vi "solar_voy_def Export (Mods_State).vi"(10 "CMD":enum8{"CMD", "TLM"}(ring), 11 "STATE":T1) -> (3 "STATE_DEF":string)   [LabVIEW 2018]
doc: "This exports a COSMOS state modifier to string."
uses:
  solar_voy_def_ctl MODIFIERS STATE.ctl
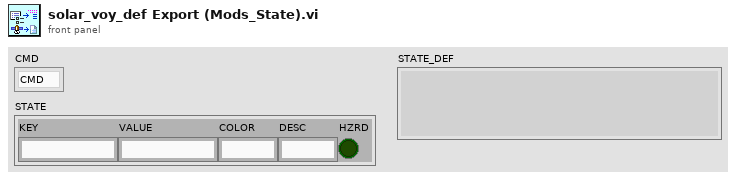
[diagram p1: front panel]
types:
  T1 = typedef "solar_voy_def_ctl MODIFIERS STATE.ctl" = cluster{"KEY":string, "VALUE":string, "COLOR":string, "DESC":string, "HZRD":bool}
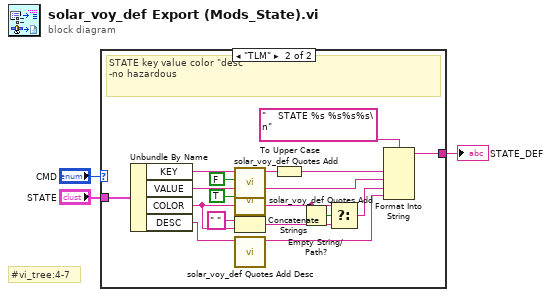
[diagram p0: block diagram]
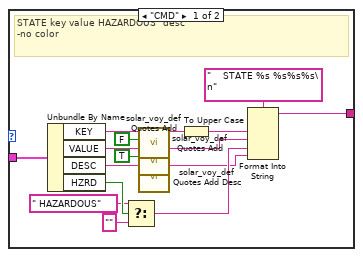
[diagram p2: hidden frame]
diagram:
  # "#vi_tree:4-7"
  n1 = case shown="\"TLM\"" "CMD" {
    tunnel: "STATE" -> [w19 w36]
    tunnel: [w12 w28] -> w2
    frame "CMD" {
      # "STATE key value HAZARDOUS \"desc\"\n-no color"
      n2 = Unbundle By Name(w19) -> ("KEY"=w17:string, "VALUE"=w16:string, "DESC"=w7:string, "HZRD"=w11:bool)
      n3 = Select(t=" HAZARDOUS", s=w11, f="") -> (s? t:f=w8:string)
      n4 = call "solar_voy_def Quotes Add.vi"("Whitespace Only? (F=Always)"=FALSE, "String"=w17) -> ("String with Comments"=w13:string)  [unwired: 9 in]
      n5 = call "solar_voy_def Quotes Add.vi"("Whitespace Only? (F=Always)"=TRUE, "String"=w16) -> ("String with Comments"=w5:string)  [unwired: 9 in]
      n6 = call "solar_voy_def Quotes Add Desc.vi"("Description"=w7) -> ("Description with Comments"=w6:string)  [unwired: 10 in]
      n7 = To Upper Case(1:w13) -> (0:w4:string)
      n8 = Format Into String(format string="    STATE %s %s%s%s\n", w4, w5, w8, w6) -> (resulting string=w12:string)  [unwired: 2 in, 1 out]
    }
    frame "TLM" {
      # "STATE key value color \"desc\"\n-no hazardous"
      n9 = Unbundle By Name(w36) -> ("KEY"=w34:string, "VALUE"=w33:string, "COLOR"=w23:string, "DESC"=w27:string)
      n10 = call "solar_voy_def Quotes Add.vi"("Whitespace Only? (F=Always)"=FALSE, "String"=w34) -> ("String with Comments"=w30:string)  [unwired: 9 in]
      n11 = call "solar_voy_def Quotes Add.vi"("Whitespace Only? (F=Always)"=TRUE, "String"=w33) -> ("String with Comments"=w29:string)  [unwired: 9 in]
      n12 = Concatenate Strings(" " ("string"), w23) -> (w22:string)
      n13 = call "solar_voy_def Quotes Add Desc.vi"("Description"=w27) -> ("Description with Comments"=w26:string)  [unwired: 10 in]
      n14 = To Upper Case(1:w30) -> (0:w20:string)
      n15 = Empty String/Path?(string/path=w23) -> (empty?=w24:bool)
      n16 = Select(t=w23, s=w24, f=w22) -> (s? t:f=w21:string)
      n17 = Format Into String(format string="    STATE %s %s%s%s\n", w20, w29, w21, w26) -> (resulting string=w28:string)  [unwired: 2 in, 1 out]
    }
  }
  "STATE_DEF" <- w2
